vi "PS Instrument UI.vi"() -> ()   [LabVIEW 2025, in "Power Supply.lvlib" / "Power Supply Instrument.lvclass"]
doc: "Copyright 2017 National Instruments Corporation\n\nLicensed under the Apache License, Version 2.0 (the \"License\"); you may not use this file except in compliance with the License. You may obtain a copy of the License at http://www.apache.org/licenses/LICENSE-2.0\nUnless required by applicable law or agreed to in writing, software distributed under the License is distributed on an \"AS IS\" BASIS, WITHOUT WARRANTIES OR CONDITIONS OF ANY KIND, either express or implied. See the License for the specific language governing permissions and limitations under the License."
uses:
  Power Supply Instrument.lvclass
  Users/Public/Documents/Sandia National Labs/TSS Plugin/CEF.lvlibp/Node/NodeRef.ctl
  Users/Public/Documents/Sandia National Labs/TSS Plugin/CEF.lvlibp/Node/CEF_Node.lvclass
  Users/Public/Documents/Sandia National Labs/TSS Plugin/CEF.lvlibp/Node/mainQref.ctl
  Users/Public/Documents/Sandia National Labs/TSS Plugin/CEF.lvlibp/Node/UserEventRef.ctl
  Users/Public/Documents/Sandia National Labs/TSS Plugin/Abstract Engine.lvlibp/Plugin/Abstract/Instrument configuration/Default Instrument.ctl
  Power Supply Instrument.lvclass/Power Supply Instrument.ctl
  <vilib>/Utility/error.llb/Trim Whitespace One-Sided.vi
  Users/Public/Documents/Sandia National Labs/TSS Plugin/Abstract Engine.lvlibp/Plugin/Abstract/Instrument configuration/Read Instrument Setting.vi
  Users/Public/Documents/Sandia National Labs/TSS Plugin/Abstract Engine.lvlibp/Plugin/Abstract/Instrument configuration/Write Instrument Setting.vi
  Users/Public/Documents/Sandia National Labs/TSS Plugin/Abstract Engine.lvlibp/Plugin/Abstract/Instrument configuration/Instrument configuration.lvclass
panel:
  in  "Power Supply":T1={"Type"="Foundation Bus", "Address"="None", "SW Alias"="None", "Description"="* Type = Class", "Enabled"=TRUE}
  in  "user event":T2
  in  "main queue":T3
  in  "node ref":T4
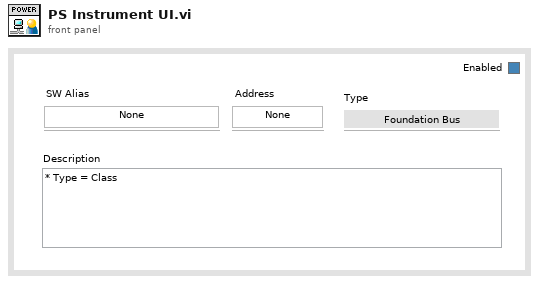
[diagram p1: front panel]
types:
  T1 = typedef "Abstract Engine.lvlibp/Instrument configuration.lvclass/Default Instrument.ctl" = cluster{"Type":string, "Address":string, "SW Alias":string, "Description":string, "Enabled":bool}
  T2 = typedef "CEF.lvlibp/CEF_Node.lvclass/UserEventRef.ctl" = refnum<user-event>
  T3 = typedef "CEF.lvlibp/CEF_Node.lvclass/mainQref.ctl" = refnum<queue>
  T4 = typedef "CEF.lvlibp/CEF_Node.lvclass/NodeRef.ctl" = refnum<data-value>
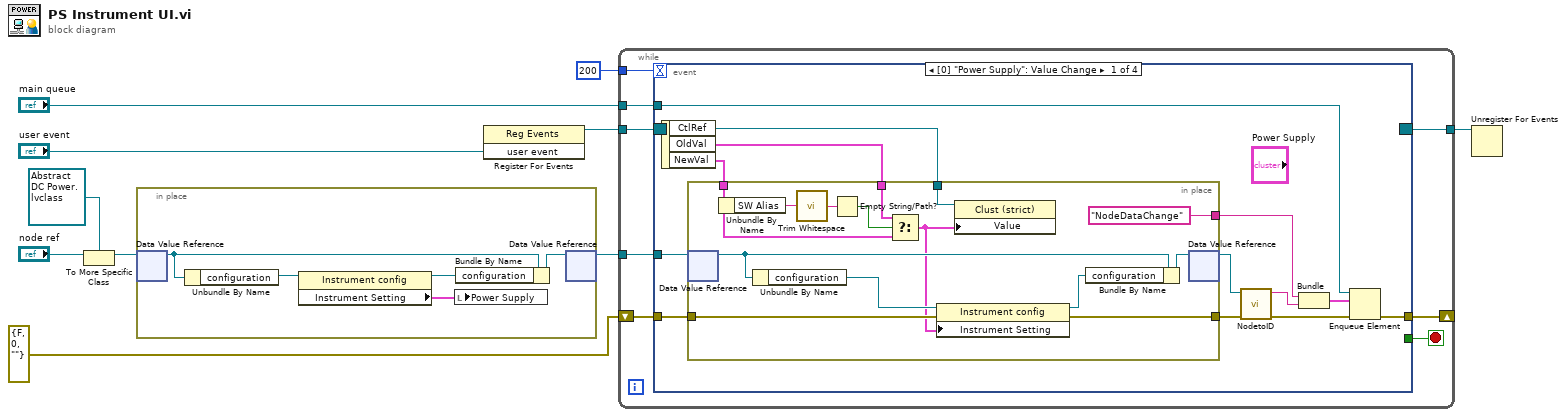
[diagram p0: block diagram]
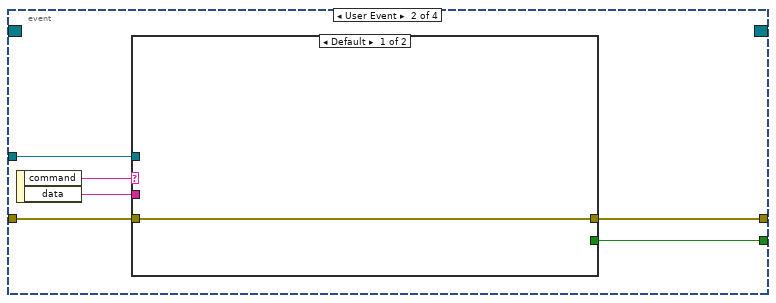
[diagram p2: hidden frame]
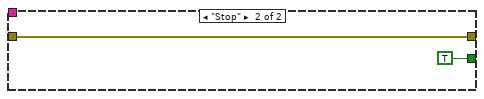
[diagram p3: hidden frame]
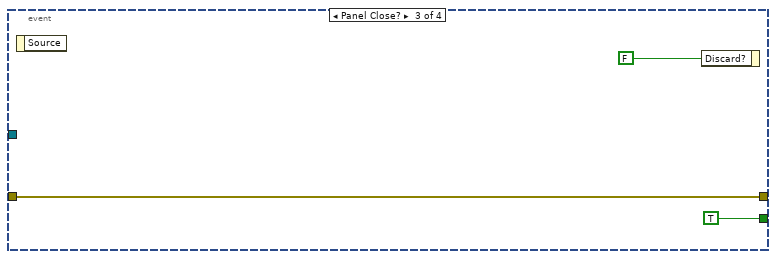
[diagram p4: hidden frame]
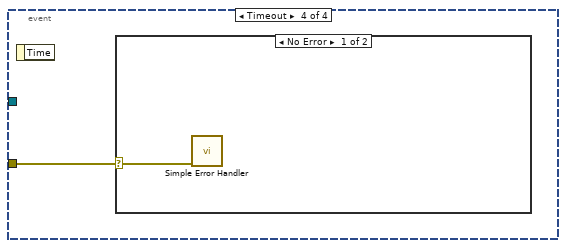
[diagram p5: hidden frame]
diagram:
  n1 = To More Specific Class(target class=refnum<data-value> refnum ("data value reference"), reference="node ref") -> (specific class reference=w3:refnum<data-value>)  [unwired: 1 in, 1 out]
  n2 = in-place {
    n3 = in-place-dvr #1(w3) -> (w12:refnum<class "Power Supply Instrument.lvclass">)  [unwired: 1 out]
    n4 = Unbundle By Name(w12) -> ("configuration"=w13:refnum<class "Instrument configuration.lvclass">)
    n5 = property class="Instrument config"(reference=w13) -> (reference out=w14:refnum<class "Instrument configuration.lvclass">, "Instrument Setting"=w11:T1)  [unwired: 1 in, 1 out]
    n6 = local write "Power Supply"(w11) -> ()
    n7 = Bundle By Name(cluster=w12, "configuration"=w14) -> (w15:refnum<class "Power Supply Instrument.lvclass">)
    n8 = in-place-dvr #1(w15) -> (w2:refnum<data-value>)  [unwired: 1 out]
  }
  n9 = register-events("user event") -> (reference out=w4:refnum<event-registration>)  [unwired: 2 in, 1 out]
  n10 = while {
    tunnel: "main queue" -> [w22]
    tunnel: w2 -> [w21]
    tunnel: w4 -> [w19]
    tunnel: [w18] -> w8
    tunnel: 200 -> [w16]
    shift-right: [w20] -> _
    shift-left: errorcluster {"status"=FALSE, "code"=0, "source"=""} ("error out") -> [w23]
    stop <- w17 stop-if-true
    n11 = event shown="[0] \"Power Supply\": Value Change" {
      selector: w19 -> [_ _ _ _]
      dyn-events: [_ _ _ _] -> w18
      timeout: w16 -> [_ _ _ _]
      tunnel: [w36 w53 w60 _] -> w20
      tunnel: w23 -> [w32 w54 w60 w63]
      tunnel: w22 -> [w35 _ _ _]
      tunnel: w21 -> [w34 w51 _ _]
      tunnel: [_ w52 TRUE _] -> w17
      event Value Change {
        n12 = event-data() -> ("CtlRef"=w29:refnum<vi>, "OldVal"=w30:T1, "NewVal"=w31:T1)  [unwired: 1 in]
        n13 = in-place {
          in-place-border: w32 -> [w49]
          in-place-border: [w47] -> w25
          in-place-border: w31 -> [w42]
          in-place-border: w30 -> [w45]
          in-place-border: w29 -> [w44]
          in-place-border: ["NodeDataChange" ("Message Name")] -> w28
          n14 = in-place-dvr #2(w34) -> (w50:refnum<class "Power Supply Instrument.lvclass">)  [unwired: 1 out]
          n15 = Unbundle By Name(w42) -> ("SW Alias"=w41:string)
          n16 = Unbundle By Name(w50) -> ("configuration"=w39:refnum<class "Instrument configuration.lvclass">)
          n17 = call <vilib>:"Trim Whitespace.vi"("string"=w41) -> ("trimmed string"=w40:string)  [unwired: 1 in]
          n18 = Empty String/Path?(string/path=w40) -> (empty?=w43:bool)
          n19 = Select(t=w45, s=w43, f=w42) -> (s? t:f=w38:T1)
          n20 = property class="Instrument config"(reference=w39, error in=w49, "Instrument Setting"=w38) -> (reference out=w46:refnum<class "Instrument configuration.lvclass">, error out=w47:errorcluster)
          n21 = property class="Clust (strict)"(reference=w44, "Value"=w38) -> ()  [unwired: 1 in, 2 out]
          n22 = Bundle By Name(cluster=w50, "configuration"=w46) -> (w48:refnum<class "Power Supply Instrument.lvclass">)
          n23 = in-place-dvr #2(w48) -> (w33:refnum<data-value>)  [unwired: 1 out]
        }
        n24 = call "NodetoID.vi"("error in"=w25, "node ref"=w33) -> ("error out"=w24:errorcluster, "ID"=w27:string)  [unwired: 8 in]
        n25 = Bundle("Message Name"=w28, "ID"=w27) -> (w26:cluster{"Message Name":string, "ID":string})  [unwired: 1 in]
        n26 = Enqueue Element(queue=w35, element=w26, error in (no error)=w24) -> (error out=w36:errorcluster)  [unwired: 1 in, 2 out]
      }
      event User Event {
        n27 = event-data() -> ("command"=w56:string, "data"=w55:string)  [unwired: 1 in]
        n28 = case shown="Default" w56 {
          tunnel: w55 -> [_ _]
          tunnel: w54 -> [w57 w59]
          tunnel: [w57 w59] -> w53
          tunnel: [_ TRUE] -> w52
          tunnel: w51 -> [_ _]
          frame Default {
          }
          frame "Stop" {
          }
        }
      }
      event Panel Close? {
        n29 = event-data() -> ()  [unwired: 1 in, 1 out]
        n30 = event-data("Discard?"=FALSE) -> ()  [unwired: 1 in, 1 out]
      }
      event Timeout {
        n31 = event-data() -> ()  [unwired: 1 in, 1 out]
        n32 = case shown="No Error" w63 {
          selector: w63 -> [w64 _]
          frame No Error {
            n33 = call <vilib>:"Simple Error Handler.vi"("error in (no error)"=w64) -> ()  [unwired: 4 in, 5 out]
          }
          frame Error {
          }
        }
      }
    }
  }
  n34 = Unregister For Events(event registration refnum=w8) -> ()  [unwired: 1 in, 1 out]
